vi "Close.vi"(0 "ACM4509 in":refnum<class "Cal Standard.lvclass">, 11 "error in (no error)":errorcluster) -> (4 "ACM4509 out":refnum<class "Cal Standard.lvclass">, 15 "error out":errorcluster)   [LabVIEW 2023, in "ACM 4509 Cal Standard.lvlib" / "Cal Standard.lvclass"]
uses:
  Cal Standard.lvclass
  Cal Standard.lvclass/Cal Standard.ctl
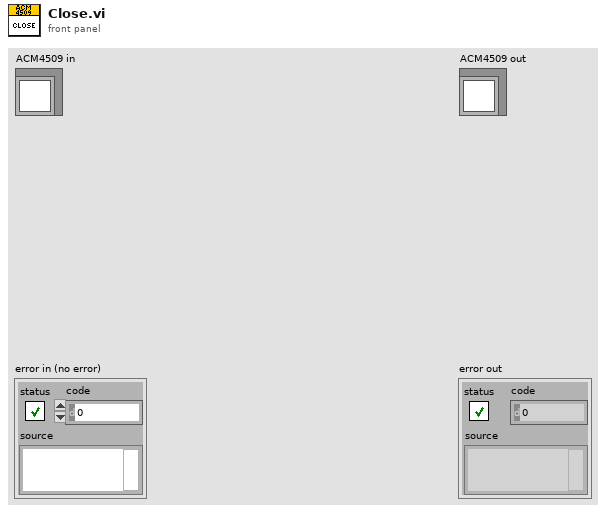
[diagram p1: front panel]
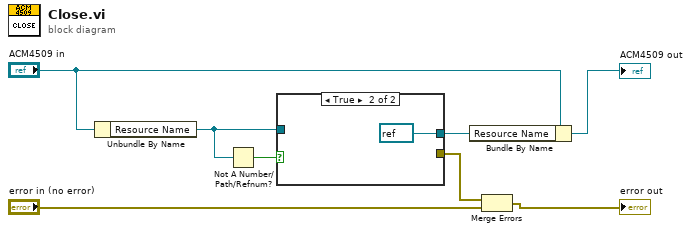
[diagram p0: block diagram]
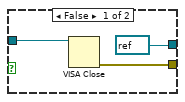
[diagram p2: hidden frame]
diagram:
  n1 = Unbundle By Name("ACM4509 in") -> ("Resource Name"=w6:refnum<visa-resource-name>)
  n2 = Not A Number/Path/Refnum?(number/path/refnum=w6) -> (NaN/Path/Refnum?=w8:bool)
  n3 = case shown="True" w8 {
    tunnel: w6 -> [w11 _]
    tunnel: [refnum<visa-resource-name> refnum ("Resource Name") refnum<visa-resource-name> refnum ("Resource Name")] -> w5
    tunnel: [w10 _] -> w7
    frame False {
      n4 = VISA Close(VISA resource name=w11) -> (error out=w10:errorcluster)  [unwired: 1 in]
    }
    frame True {
    }
  }
  n5 = Bundle By Name(cluster="ACM4509 in", "Resource Name"=w5) -> (→"ACM4509 out":refnum<class "Cal Standard.lvclass">)
  n6 = Merge Errors(w7, "error in (no error)") -> (→"error out":errorcluster)
